vi "Cursors4Contrast.vi"(2 "Bound 2":dbl, 3 "Bound 1":dbl, 4 "Second array":dbl[][](array[numeric]), 5 "Array to search":dbl[](array[numeric])) -> (0 "Second array reduced by bounds":dbl[][](array[numeric]), 1 "Array reduced by bounds":dbl[](array[numeric]))   [LabVIEW 2019]
panel:
  out "Index bound 1 real":dbl
  out "Index bound 2 real":dbl
  out "size(s)":i32
  out "Index bound 2":dbl
  out "Index bound 1":dbl
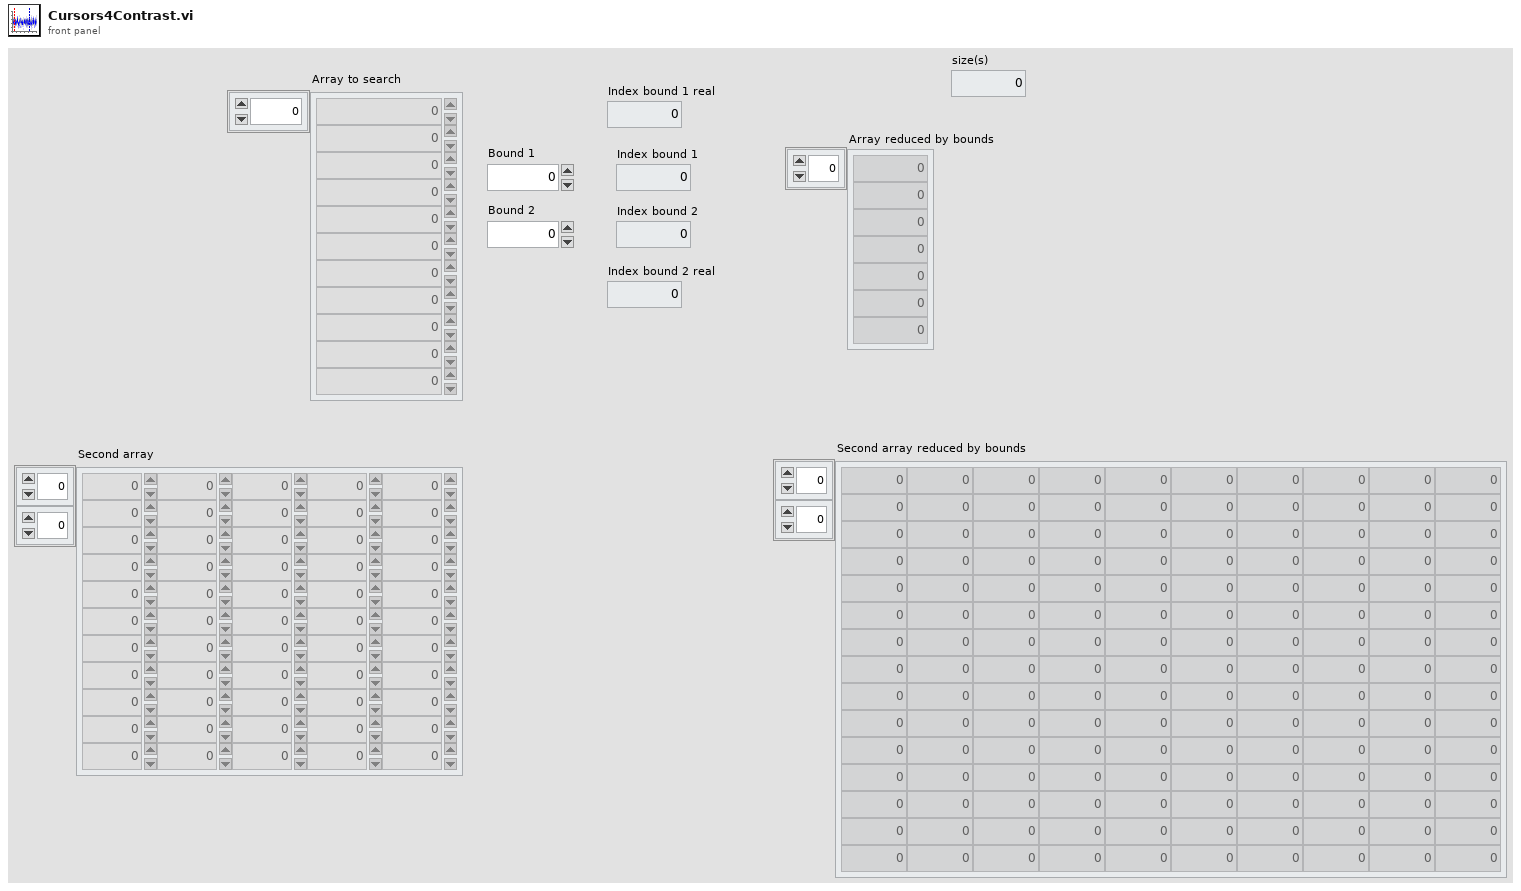
[diagram p1: front panel]
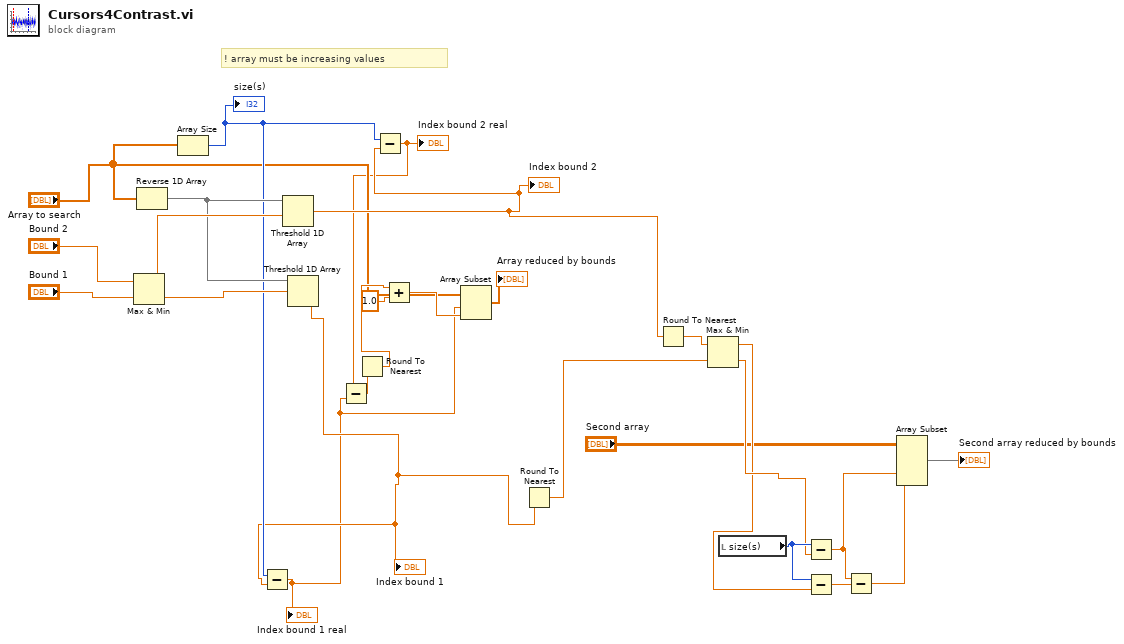
[diagram p0: block diagram]
diagram:
  # "! array must be increasing values"
  n1 = Max & Min(x="Bound 2", y="Bound 1") -> (max(x,y)=w19:dbl, min(x,y)=w20:dbl)
  n2 = Reverse 1D Array(array="Array to search") -> (reversed array=w18:dbl[])
  n3 = Array Size(array="Array to search") -> (size(s)=w5:i32)
  "size(s)" <- w5
  n4 = Threshold 1D Array(2:w19, 3:w18) -> (0:w6:dbl)  [unwired: 1 in]
  "Index bound 2" <- w6
  n5 = Threshold 1D Array(2:w20, 3:w18) -> (0:w4:dbl)  [unwired: 1 in]
  "Index bound 1" <- w4
  n6 = Subtract(x=w5, y=w4) -> (x-y=w1:dbl)
  "Index bound 1 real" <- w1
  n7 = Subtract(x=w5, y=w6) -> (x-y=w2:dbl)
  "Index bound 2 real" <- w2
  n8 = Subtract(x=w2, y=w1) -> (x-y=w17:dbl)
  n9 = Round To Nearest(number=w17) -> (nearest integer value=w16:dbl)
  n10 = Add(x=w16, y=1.0) -> (x+y=w21:dbl)
  n11 = Array Subset(array="Array to search", index=w1, length=w21) -> (→"Array reduced by bounds":dbl[])
  n12 = Round To Nearest(number=w4) -> (nearest integer value=w14:dbl)
  n13 = Round To Nearest(number=w6) -> (nearest integer value=w15:dbl)
  n14 = Max & Min(x=w15, y=w14) -> (max(x,y)=w11:dbl, min(x,y)=w12:dbl)
  n15 = local read "size(s)"() -> (w13:i32)
  n16 = Subtract(x=w13, y=w12) -> (x-y=w8:dbl)
  n17 = Subtract(x=w13, y=w11) -> (x-y=w9:dbl)
  n18 = Subtract(x=w8, y=w9) -> (x-y=w10:dbl)
  n19 = Array Subset(array="Second array", index (col)=w8, length (col)=w10) -> (→"Second array reduced by bounds":dbl[][])  [unwired: 2 in]
